vi "Settings_dialog.vi"(11 "Options":T1={"Form_data_log_period"=0, "startup_threshold"=0.0, "Coeff_U"=2.55, "Offset_U"=6.5, "Coeff_I"=42.391, "Offset_I"=77.0, "Save_data_path"=path "", "ADC_frequency"=50000.0, "VISA resource name"="COM1"} caption="Настройки") -> (1 "Canceled":bool, 3 "Options_out":T1={"Form_data_log_period"=0, "startup_threshold"=0.0, "Coeff_U"=2.55, "Offset_U"=6.5, "Coeff_I"=42.391, "Offset_I"=77.0, "Save_data_path"=path "", "ADC_frequency"=50000.0, "VISA resource name"="COM1"})   [LabVIEW 2012]
uses:
  Controls/options.ctl
panel:
  in  "Apply options":bool
  in  "Cancel options":bool
  # "с"
  # "В"
  # "Настройки АЦП"
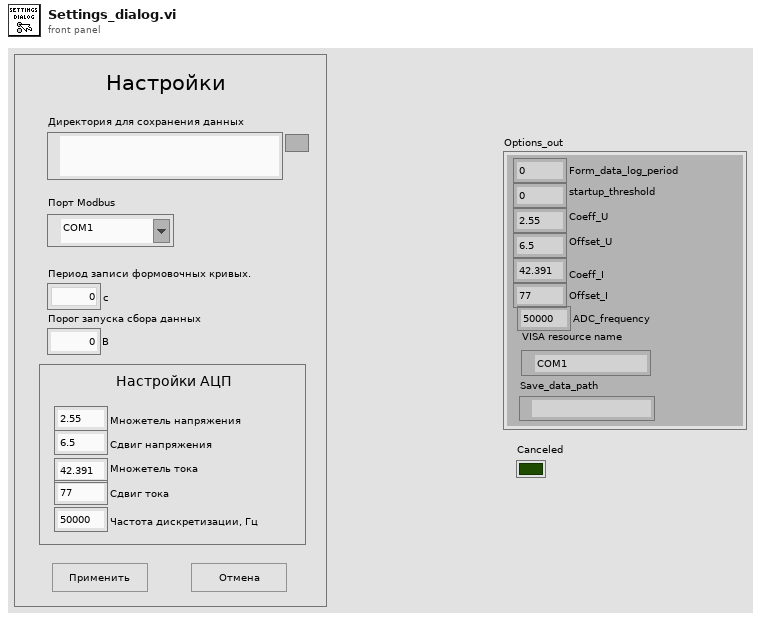
[diagram p1: front panel]
types:
  T1 = typedef "options.ctl" = cluster{"Form_data_log_period":i32, "startup_threshold":dbl, "Coeff_U":dbl, "Offset_U":dbl, "Coeff_I":dbl, "Offset_I":dbl, "Save_data_path":path, "ADC_frequency":dbl, "VISA resource name":refnum<visa-resource-name>}
  T2 = enum32{"Invalid", "Standard", "Closed", "Hidden", "Minimized", "Maximized"}
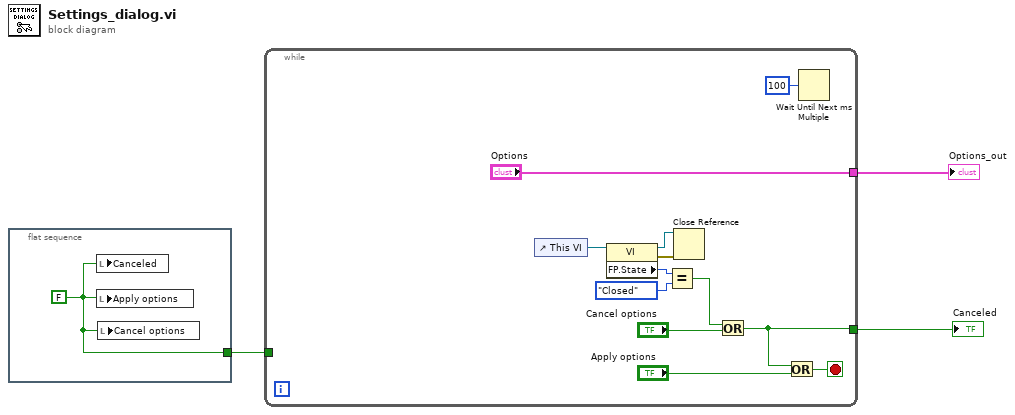
[diagram p0: block diagram]
diagram:
  n1 = flat-sequence {
    tunnel: [w4] -> w3
    frame #0 {
      w4 = FALSE
      n2 = local write "Canceled"(w4) -> ()
      n3 = local write "Apply options"(w4) -> ()
      n4 = local write "Cancel options"(w4) -> ()
    }
  }
  n5 = while {
    tunnel: w3 -> [_]
    tunnel: ["Options"] -> w2
    tunnel: [w6] -> w1
    stop <- w16 stop-if-true
    n6 = control-ref of="This VI"() -> (w13:refnum<vi>)
    n7 = property class="VI"(reference=w13) -> (reference out=w11:refnum<vi>, error out=w12:errorcluster, "FP.State"=w10:T2)  [unwired: 1 in]
    n8 = Equal?(x=w10, y=T2."Closed" ("Front Panel Window:State")) -> (x = y?=w7:bool)
    n9 = Close Reference(reference=w11, error in (no error)=w12) -> ()  [unwired: 1 out]
    n10 = Or(x=w7, y="Cancel options") -> (x .or. y?=w6:bool)
    n11 = Or(x=w6, y="Apply options") -> (x .or. y?=w16:bool)
    n12 = Wait Until Next ms Multiple(millisecond multiple=u32 100) -> ()  [unwired: 1 out]
  }
  "Canceled" <- w1
  "Options_out" <- w2
